vi "Thread@MutePopupMessage__Parameter.vi"(1 "ParamterIn":string) -> (0 "ParamterOut":string)   [LabVIEW 2020]
panel:
  in  "Mute":string(combo)="1"
  in  "Confirm":bool
  # "Thread@MutePopupMessage {0,1}"
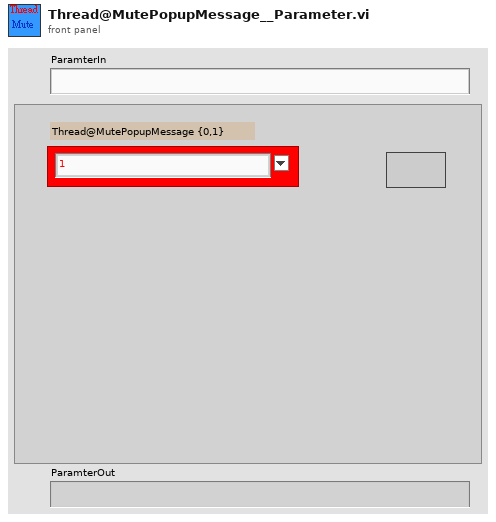
[diagram p1: front panel]
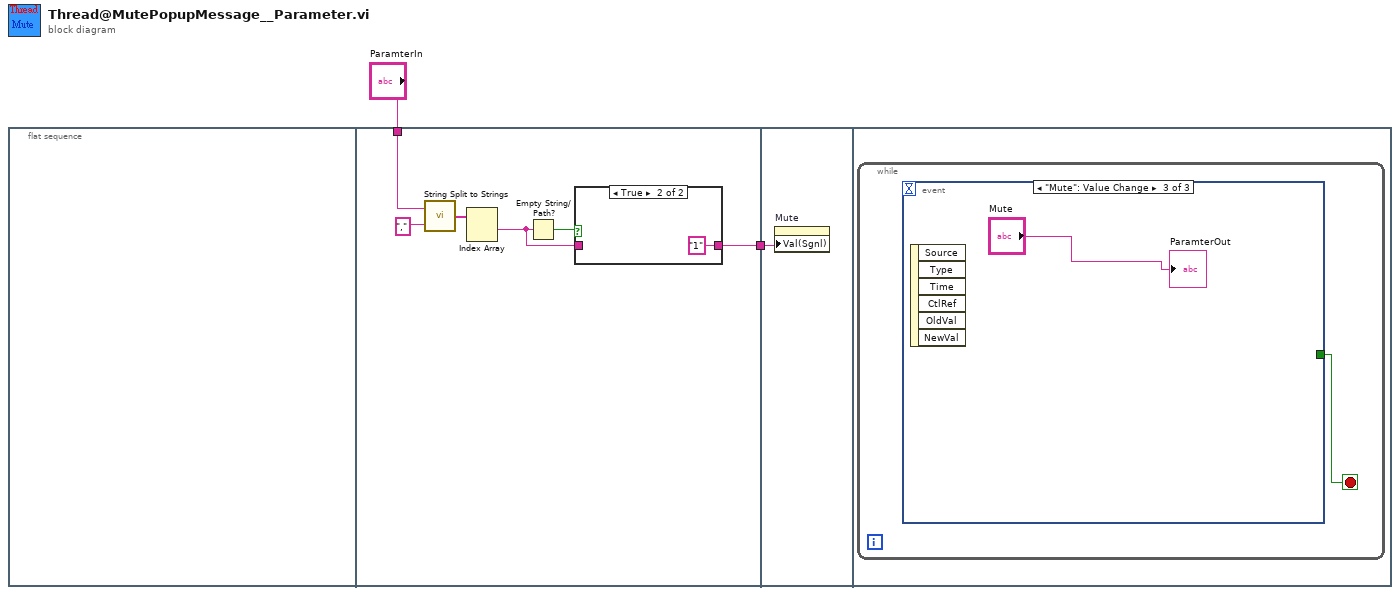
[diagram p0: block diagram]
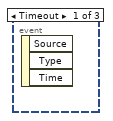
[diagram p3: hidden frame]
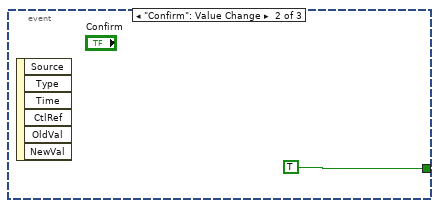
[diagram p4: hidden frame]
diagram:
  n1 = flat-sequence {
    tunnel: "ParamterIn" -> [w6]
    tunnel: [w3] -> w1
    tunnel: w1 -> [w11]
    frame #0 {
    }
    frame #1 {
      n2 = call "String Split to Strings.vi"("search string/char (-)"=",", "String"=w6) -> ("Array"=w8:string[])
      n3 = Index Array(array=w8) -> (element #1=w4:string)  [unwired: 2 in, 1 out]
      n4 = Empty String/Path?(string/path=w4) -> (empty?=w5:bool)
      n5 = case shown="True" w5 {
        tunnel: w4 -> [w9 _]
        tunnel: [w9 "1"] -> w3
        frame False {
        }
        frame True {
        }
      }
    }
    frame #2 {
      n6 = property on="Mute" class="CmbBox"("Val(Sgnl)"=w11) -> ()  [unwired: 2 in, 2 out]
    }
    frame #3 {
      n7 = while {
        stop <- w12 stop-if-true
        n8 = event shown="[2] \"Mute\": Value Change" {
          selector: _ -> [_ _ _]
          dyn-events: _ -> [_ _ _]
          timeout: _ -> [_ _ _]
          tunnel: [_ TRUE _] -> w12
          event Timeout {
            n9 = event-data() -> ()  [unwired: 1 in, 3 out]
          }
          event "Confirm": Value Change {
            n10 = event-data() -> ()  [unwired: 1 in, 6 out]
          }
          event "Mute": Value Change {
            n11 = event-data() -> ()  [unwired: 1 in, 6 out]
            "ParamterOut" <- "Mute"
          }
        }
      }
    }
  }
